vi "RTS MX Data Parse.vi"(7 "System Number":T1="Sys1", 8 "Error In":errorcluster, 11 "Input Data":string[][](array[string])) -> (0 "Error Out":errorcluster, 3 "Output Data":string[][](array[string]))   [LabVIEW 2016]
uses:
  Type Definitions/RTS Select System Number.ctl
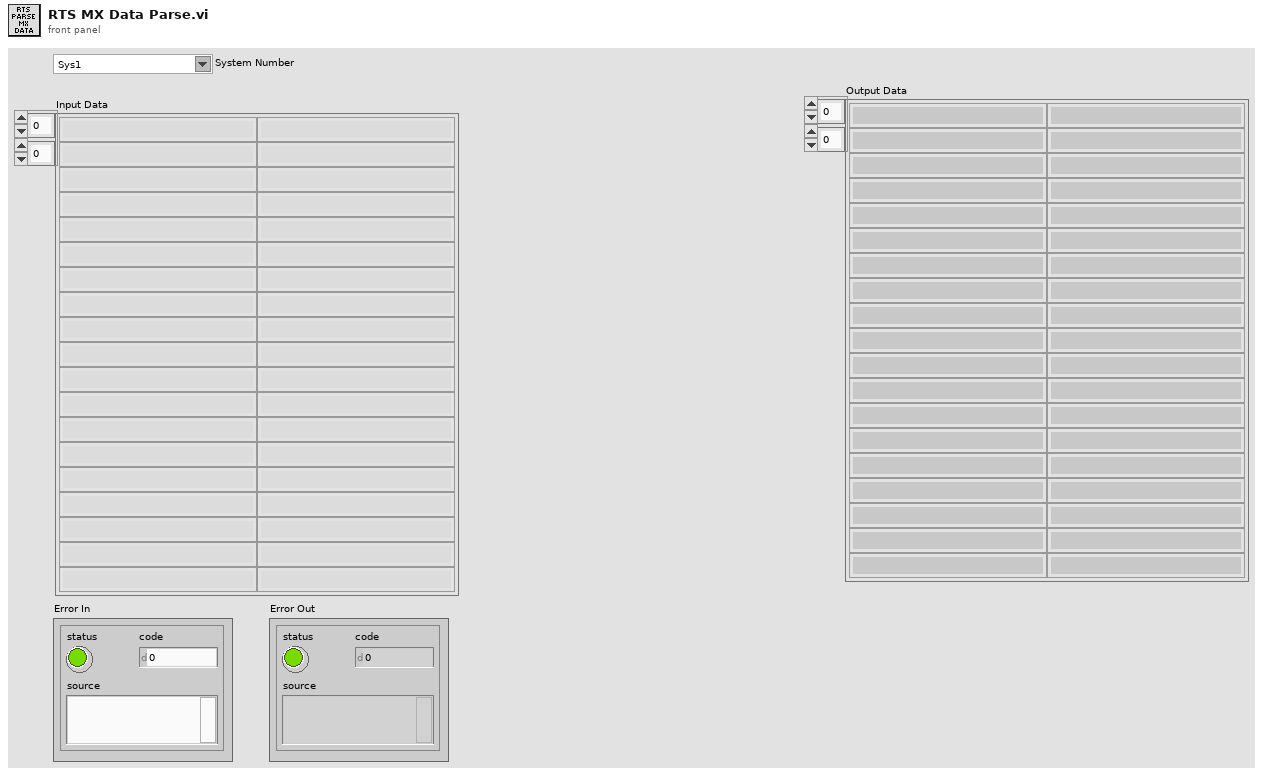
[diagram p1: front panel]
types:
  T1 = typedef "RTS Select System Number.ctl" = string
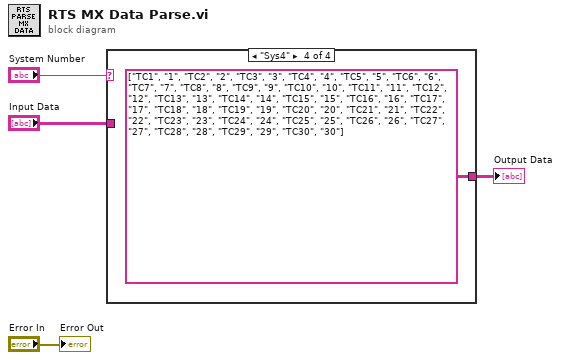
[diagram p0: block diagram]
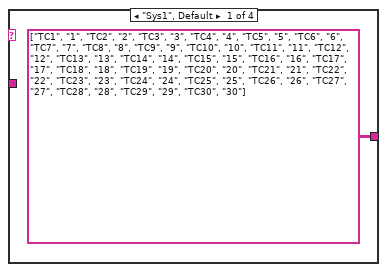
[diagram p2: hidden frame]
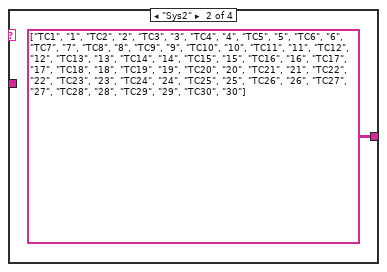
[diagram p3: hidden frame]
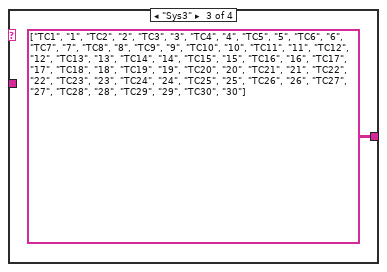
[diagram p4: hidden frame]
diagram:
  n1 = case shown="\"Sys4\"" "System Number" {
    tunnel: "Input Data" -> [_ _ _ _]
    tunnel: [string[][] [["TC1", "1"], ["TC2", "2"], ["TC3", "3"], ["TC4", "4"], ["TC5", "5"], ["TC6", "6"], ["TC7", "7"], ["TC8", "8"], ["TC9", "9"], ["TC10", "10"], ["TC11", "11"], ["TC12", "12"], ["TC13", "13"], ["TC14", "14"], ["TC15", "15"], ["TC16", "16"], ["TC17", "17"], ["TC18", "18"], ["TC19", "19"], ["TC20", "20"], ["TC21", "21"], ["TC22", "22"], ["TC23", "23"], ["TC24", "24"], ["TC25", "25"], ["TC26", "26"], ["TC27", "27"], ["TC28", "28"], ["TC29", "29"], ["TC30", "30"]] ("Input Data") string[][] [["TC1", "1"], ["TC2", "2"], ["TC3", "3"], ["TC4", "4"], ["TC5", "5"], ["TC6", "6"], ["TC7", "7"], ["TC8", "8"], ["TC9", "9"], ["TC10", "10"], ["TC11", "11"], ["TC12", "12"], ["TC13", "13"], ["TC14", "14"], ["TC15", "15"], ["TC16", "16"], ["TC17", "17"], ["TC18", "18"], ["TC19", "19"], ["TC20", "20"], ["TC21", "21"], ["TC22", "22"], ["TC23", "23"], ["TC24", "24"], ["TC25", "25"], ["TC26", "26"], ["TC27", "27"], ["TC28", "28"], ["TC29", "29"], ["TC30", "30"]] ("Input Data") string[][] [["TC1", "1"], ["TC2", "2"], ["TC3", "3"], ["TC4", "4"], ["TC5", "5"], ["TC6", "6"], ["TC7", "7"], ["TC8", "8"], ["TC9", "9"], ["TC10", "10"], ["TC11", "11"], ["TC12", "12"], ["TC13", "13"], ["TC14", "14"], ["TC15", "15"], ["TC16", "16"], ["TC17", "17"], ["TC18", "18"], ["TC19", "19"], ["TC20", "20"], ["TC21", "21"], ["TC22", "22"], ["TC23", "23"], ["TC24", "24"], ["TC25", "25"], ["TC26", "26"], ["TC27", "27"], ["TC28", "28"], ["TC29", "29"], ["TC30", "30"]] ("Input Data") string[][] [["TC1", "1"], ["TC2", "2"], ["TC3", "3"], ["TC4", "4"], ["TC5", "5"], ["TC6", "6"], ["TC7", "7"], ["TC8", "8"], ["TC9", "9"], ["TC10", "10"], ["TC11", "11"], ["TC12", "12"], ["TC13", "13"], ["TC14", "14"], ["TC15", "15"], ["TC16", "16"], ["TC17", "17"], ["TC18", "18"], ["TC19", "19"], ["TC20", "20"], ["TC21", "21"], ["TC22", "22"], ["TC23", "23"], ["TC24", "24"], ["TC25", "25"], ["TC26", "26"], ["TC27", "27"], ["TC28", "28"], ["TC29", "29"], ["TC30", "30"]] ("Input Data")] -> w1
    frame "Sys1", Default {
    }
    frame "Sys2" {
    }
    frame "Sys3" {
    }
    frame "Sys4" {
    }
  }
  "Output Data" <- w1
  "Error Out" <- "Error In"
